vi "XYStage.OnMoveCompleted.vi"(8 "error in (no error)":errorcluster, 10 "Move Completed":T1, 11 "XYStage":refnum<class "XYStage.lvclass">) -> (0 "error out":errorcluster, 3 "XYStage out":refnum<class "XYStage.lvclass">)   [LabVIEW 2017, in "XYStage.lvclass"]
doc: "---------------------------------------------------------------\nJKI State Machine Objects™\nhttp://jki.net/state-machine-objects/\nCopyright (C) 2005-2015, JKI <info@jki.net>\nALL RIGHTS RESERVEDJKI State Machine Objects (SMO) 1.0.0.4\nJKI - JKI\nCopyright (c) 2015, JKI"
uses:
  XYStage.lvclass
  Typedefs/PublicEvents--XYStage.MoveCompleted.ctl
  Typedefs/Coordinates--Cluster.ctl
  Typedefs/Coordinates.Units--Cluster.ctl
  Typedefs/Coordinates.Counts--Cluster.ctl
  XYStage.lvclass/XYStage.ctl
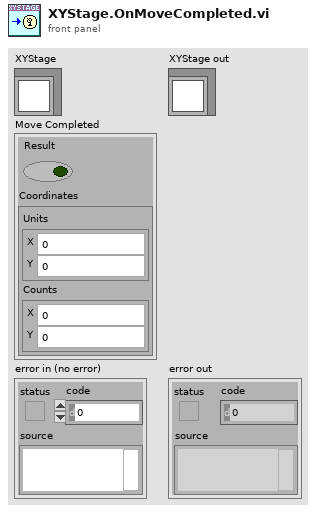
[diagram p1: front panel]
types:
  T1 = typedef "XYStage.lvclass/PublicEvents--XYStage.MoveCompleted.ctl" = cluster{"Result":bool, "Coordinates":T2}
  T2 = typedef "XYStage.lvclass/Coordinates--Cluster.ctl" = cluster{"Units":T3, "Counts":T4}
  T3 = typedef "XYStage.lvclass/Coordinates.Units--Cluster.ctl" = cluster{"X":dbl, "Y":dbl}
  T4 = typedef "XYStage.lvclass/Coordinates.Counts--Cluster.ctl" = cluster{"X":i32, "Y":i32}
  T5 = typedef "XYStage.lvclass/PrivateData--Ref.ctl" = refnum<data-value>
  T6 = typedef "XYStage.lvclass/PrivateData--Cluster.ctl" = cluster{"Configuration":T7, "Public Events":T8, "Protected Events":T9, "Private Events":T10}
  T7 = typedef "XYStage.lvclass/Configuration--Cluster.ctl" = cluster{"Serial Number":string, "X Axis":string, "Y Axis":string, "Real-World Units":string, "Counts per Unit":u32}
  T8 = typedef "XYStage.lvclass/PublicEvents--Cluster.ctl" = cluster{"MoveStarted":refnum<user-event>, "MoveCompleted":refnum<user-event>}
  T9 = typedef "XYStage.lvclass/ProtectedEvents--Cluster.ctl" = cluster{"StatusUpdated":refnum<user-event>}
  T10 = typedef "XYStage.lvclass/PrivateEvents--Cluster.ctl" = cluster{"MoveAbsolute (units)":refnum<user-event>}
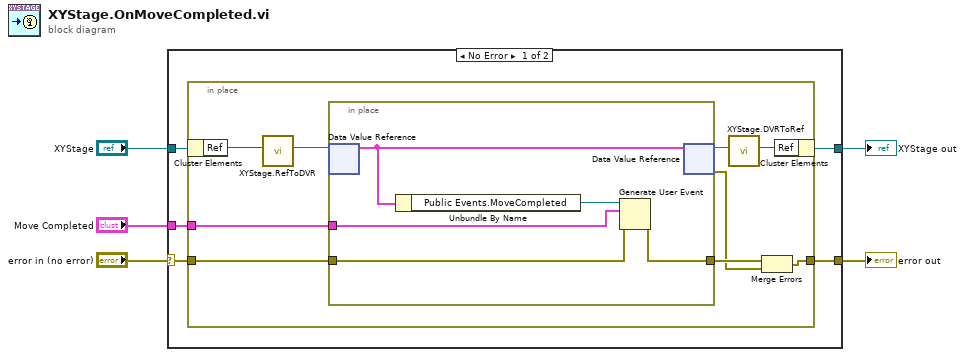
[diagram p0: block diagram]
diagram:
  n1 = case shown="No Error" "error in (no error)" {
    selector: "error in (no error)" -> [w8 w26]
    tunnel: [w7 w26] -> w4
    tunnel: [w9 w25] -> w5
    tunnel: "XYStage" -> [w10 w25]
    tunnel: "Move Completed" -> [w6 _]
    frame No Error {
      n2 = in-place {
        in-place-border: w8 -> [w19]
        in-place-border: [w16] -> w7
        in-place-border: w6 -> [w11]
        n3 = in-place-cluster #1(w10) -> ("Ref"=w15:u32)
        n4 = call "XYStage.RefToDVR.vi"("Ref"=w15) -> ("Ref"=w13:T5)  [unwired: 10 in]
        n5 = in-place {
          in-place-border: w19 -> [w22]
          in-place-border: [w21] -> w18
          in-place-border: w11 -> [w20]
          n6 = in-place-dvr #2(w13) -> (w24:T6)  [unwired: 1 out]
          n7 = Unbundle By Name(w24) -> ("Public Events.MoveCompleted"=w23:refnum<user-event>)
          n8 = Generate User Event(user event=w23, event data cluster=w20, error in=w22) -> (error out=w21:errorcluster)  [unwired: 1 in, 1 out]
          n9 = in-place-dvr #2(w24) -> (w14:T5, w17:errorcluster)
        }
        n10 = call "XYStage.DVRToRef.vi"("Ref"=w14) -> ("Ref"=w12:u32)  [unwired: 10 in]
        n11 = Merge Errors(w18, w17) -> (w16:errorcluster)
        n12 = in-place-cluster #1("Ref"=w12) -> (w9:refnum<class "XYStage.lvclass">)
      }
    }
    frame Error {
    }
  }
  "error out" <- w4
  "XYStage out" <- w5
